vi "parse_dataframe.vi"(11 "dataframe":string) -> (3 "DataFrame.lvclass":refnum<class "DataFrame.lvclass">)   [LabVIEW 2017, in "DataFrame.lvclass"]
uses:
  DataFrame.lvclass
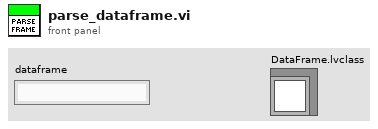
[diagram p1: front panel]
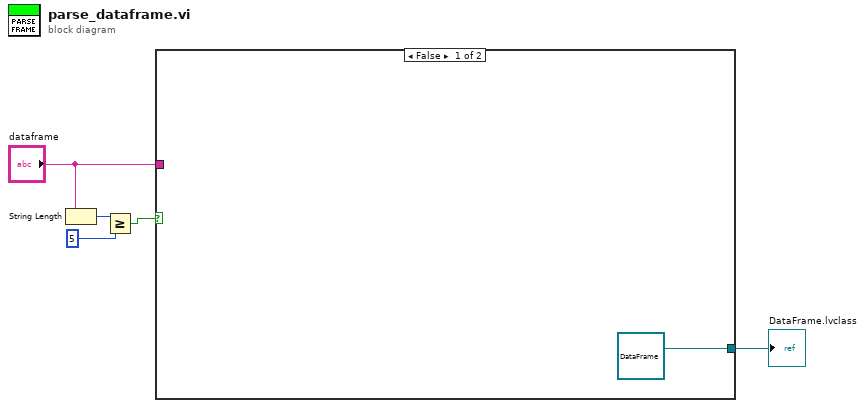
[diagram p0: block diagram]
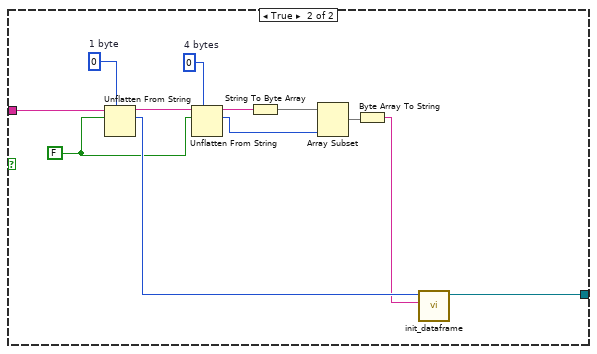
[diagram p2: hidden frame]
diagram:
  n1 = String Length(string="dataframe") -> (length=w4:i32)
  n2 = Greater Or Equal?(x=w4, y=5) -> (x >= y?=w2:bool)
  n3 = case shown="False" w2 {
    tunnel: "dataframe" -> [_ w8]
    tunnel: [refnum<class "DataFrame.lvclass"> refnum ("DataFrame.lvclass") w7] -> w1
    frame False {
    }
    frame True {
      w16 = u32 0  # 4 bytes
      w18 = u8 0  # 1 byte
      w14 = FALSE ("data includes array or string size? (T)")
      n4 = Unflatten From String(type=w18, binary string=w8, data includes array or string size? (T)=w14) -> (rest of the binary string=w17:string, value=w15:u8)  [unwired: 2 in, 1 out]
      n5 = Unflatten From String(type=w16, binary string=w17, data includes array or string size? (T)=w14) -> (rest of the binary string=w13:string, value=w11:u32)  [unwired: 2 in, 1 out]
      n6 = String To Byte Array(string=w13) -> (unsigned byte array=w12:u8[])
      n7 = Array Subset(array=w12, length=w11) -> (w10:u8[])  [unwired: 1 in]
      n8 = Byte Array To String(unsigned byte array=w10) -> (string=w9:string)
      n9 = call "init_dataframe.vi"("data"=w9, "command type"=w15) -> ("DataFrame.lvclass"=w7:refnum<class "DataFrame.lvclass">)  [unwired: 9 in]
    }
  }
  "DataFrame.lvclass" <- w1
